vi "Configure DAQ Trigger (Marker0 to Ctr).vi"(8 "error in (no error)":errorcluster, 9 "FGEN Channels":string[](array[string]), 10 "FGEN Resource":refnum<k15>, 11 "DAQmx Tasks In":T2) -> (0 "error out":errorcluster, 2 "FGEN-DAQ Routing":T1, 3 "DAQmx Tasks Out":T2)   [LabVIEW 2025]
uses:
  <vilib>/DAQmx/configure/trigger.llb/DAQmx Start Trigger (Digital Edge).vi
  <resource>/objmgr/daqmx.rc
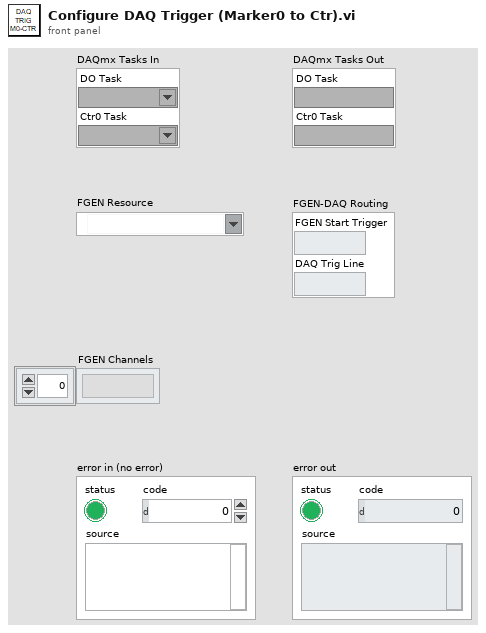
[diagram p1: front panel]
types:
  T1 = cluster{"FGEN Start Trigger":string, "DAQ Trig Line":string}
  T2 = cluster{"DO Task":refnum<k21>, "Ctr0 Task":refnum<k21>}
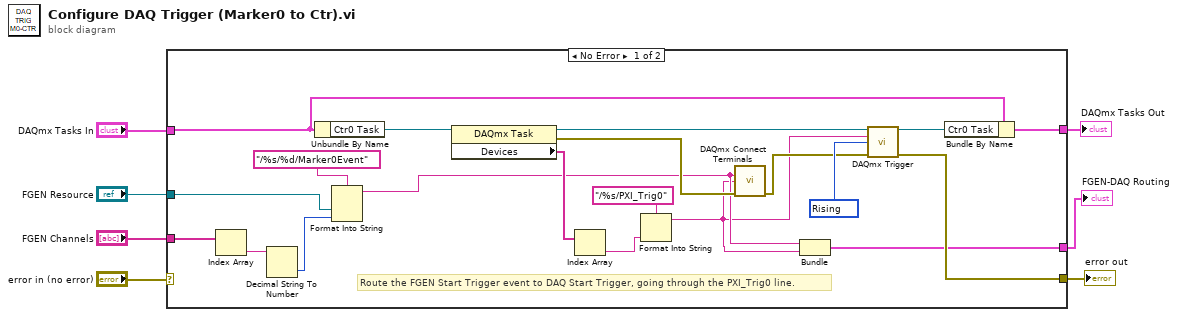
[diagram p0: block diagram]
diagram:
  n1 = case shown="No Error" "error in (no error)" {
    selector: "error in (no error)" -> [_ w28]
    tunnel: [w19 w28] -> w7
    tunnel: "DAQmx Tasks In" -> [w17 _]
    tunnel: [w18 _] -> w4
    tunnel: "FGEN Resource" -> [w24 _]
    tunnel: "FGEN Channels" -> [w25 _]
    tunnel: [w8 _] -> w1
    frame No Error {
      w21 = 10280 items=["Rising"=10280, "Falling"=10171] ("edge")
      # "Route the FGEN Start Trigger event to DAQ Start Trigger, going through the PXI_Trig0 line."
      n2 = Index Array(array=w25) -> (element=w23:string)  [unwired: 1 in]
      n3 = Decimal String To Number(string=w23) -> (number=w22:i32)  [unwired: 2 in, 1 out]
      n4 = Unbundle By Name(w17) -> ("Ctr0 Task"=w20:refnum<k21>)
      n5 = Format Into String(format string="/%s/%d/Marker0Event", w24, w22) -> (resulting string=w10:string)  [unwired: 2 in, 1 out]
      n6 = property class="DAQmx Task"(reference=w20) -> (reference out=w16:refnum<k21>, error out=w12:errorcluster, "Devices"=w15:tag[])  [unwired: 1 in]
      n7 = Index Array(array=w15) -> (element=w13:tag)  [unwired: 1 in]
      n8 = Format Into String(format string="/%s/PXI_Trig0", w13) -> (resulting string=w9:string)  [unwired: 2 in, 1 out]
      n9 = call <vilib>:"DAQmx Connect Terminals.vi"("source terminal"=w10, "destination terminal"=w9, "error in"=w12) -> ("error out"=w11:errorcluster)  [unwired: 12 in]
      n10 = Bundle(w10, w9) -> (w8:cluster{string, string})  [unwired: 1 in]
      n11 = call-poly <vilib>:"DAQmx Trigger.vi"("task/channels in"=w16, "source"=w9, "edge"=w21, "error in"=w11) -> ("task out"=w27:refnum<k21>, "error out"=w19:errorcluster)  [unwired: 10 in]
      n12 = Bundle By Name(cluster=w17, "Ctr0 Task"=w27) -> (w18:T2)
    }
    frame Error {
    }
  }
  "error out" <- w7
  "DAQmx Tasks Out" <- w4
  "FGEN-DAQ Routing" <- w1
